vi "Scale 2D.vi"(0 "X":dbl[][](array[numeric]) format="%0.2f") -> (1 "Y=(X-offset)/scale":dbl[][](array[numeric]) format="%0.2f", 2 "scale":dbl format="%0.2f", 3 "offset":dbl format="%0.2f", 4 "error":i32)   [LabVIEW 2017, in "NI_AALBase.lvlib"]
doc: "Removes the <B>offset</B> of an input signal <B>X</B> and then scales the result so that the output sequence is in the range [-1:1]."
uses:
  NI_AALBase.lvlib
  lvanlys.dll
panel:
  # "Yij=(Xij-offset)/scale"
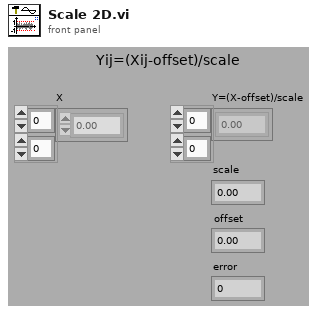
[diagram p1: front panel]
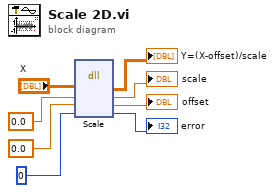
[diagram p0: block diagram]
diagram:
  n1 = dll-call lib="C:/Program Files/National Instruments/LabVIEW 2017/resource/lvanlys.*" fn="Scale"("X"="X", 0.0, 0.0, 0) -> ("X"=→"Y=(X-offset)/scale":dbl[][], →"scale":dbl, →"offset":dbl, →"error":i32)  [unwired: 4 in, 2 out]
